vi "Sweep.vi"(0 "LINX Resource":T1, 5 "Bias V":dbl, 7 "steps to record":i32, 11 "error in (no error)":errorcluster) -> (4 "LINX Resource 2":T1, 6 "PD current (A)":dbl[](array[numeric]), 8 "Incidence angle (deg)":dbl[](array[numeric]), 10 "PD Voltage (V)":dbl[](array[numeric]), 15 "Error Out":errorcluster)   [LabVIEW 2020]
uses:
  <vilib>/MakerHub/LINX/Private/Type Defs/LINX Ref.ctl
  <vilib>/MakerHub/LINX/Private/Type Defs/Platform.ctl
  <vilib>/MakerHub/LINX/Private/Type Defs/Interface.ctl
  <vilib>/MakerHub/LINX/Private/Device/Type Defs/LINX Device Config.ctl
  <vilib>/MakerHub/LINX/Private/Device/Type Defs/TCP Config.ctl
  <vilib>/MakerHub/LINX/Private/Device/Type Defs/Channels.ctl
  <vilib>/MakerHub/LINX/Public/Peripherals/Digital/Digital Write 1 Chan.vi
  <vilib>/MakerHub/LINX/Public/Peripherals/Digital/Digital Write N Chans.vi
  <vilib>/MakerHub/LINX/Private/Local IO/LinxDigitalWrite.vi
  <vilib>/MakerHub/LINX/Public/Utilities/Check Channel.vi
  <vilib>/MakerHub/LINX/Private/Utilties/Generate Error.vi
  <vilib>/MakerHub/LINX/LMH-LINX.lvlib
  <vilib>/MakerHub/LINX/Private/Device/Device.lvlib
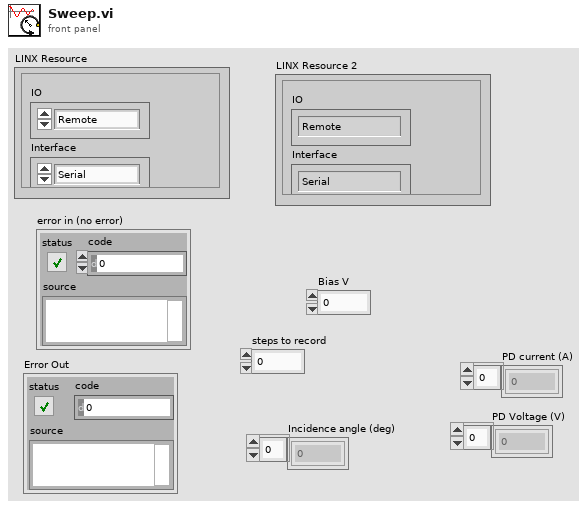
[diagram p1: front panel]
types:
  T1 = typedef "LMH-LINX.lvlib/LINX Ref.ctl" = cluster{"IO":T2, "Interface":T3, "LINX Device Config":T4}
  T2 = typedef "LMH-LINX.lvlib/Platform.ctl" = enum16{"Remote", "Local"}
  T3 = typedef "LMH-LINX.lvlib/Interface.ctl" = enum16{"Serial", "TCP"}
  T4 = typedef "LMH-LINX.lvlib/Device.lvlib/LINX Device Config.ctl" = cluster{"Interface":T3, "COM Port":refnum<visa-resource-name>, "TCP Configuration":T5, "Device Family":u8, "Device ID":u8, "Device Name":string, "TCP Ref":refnum<k5>, "Channels":T6}
  T5 = typedef "LMH-LINX.lvlib/Device.lvlib/TCP Config.ctl" = cluster{"IP Address":string, "Port":u16}
  T6 = typedef "LMH-LINX.lvlib/Channels.ctl" = cluster{"DI":u8[], "DO":u8[], "AI":u8[], "AO":u8[], "PWM":u8[], "QE":u8[], "UART":u8[], "I2C 2":u8[], "SPI":u8[], "CAN":u8[], "Servo":u8[], "AI Ref (V)":dbl, "AI Resolution (Bits)":u8, "AO Ref (V)":dbl, "AO Resolution (Bits)":u8}
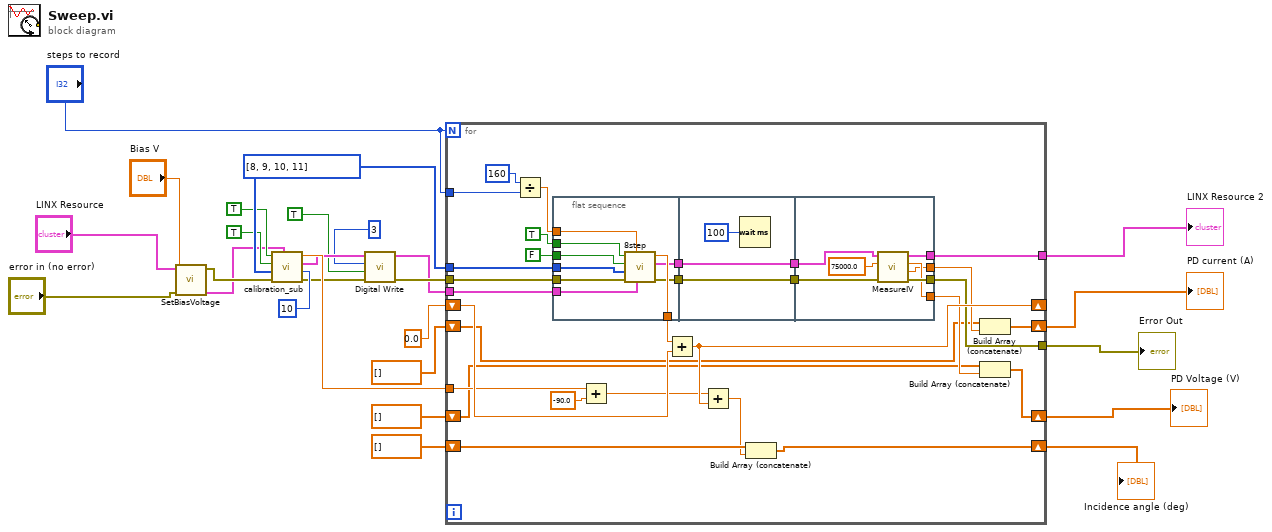
[diagram p0: block diagram]
diagram:
  w26 = u8[] [8, 9, 10, 11] ("DO Channels")
  n1 = call "SetBiasVoltage.vi"("Error In"="error in (no error)", "Bias V"="Bias V", "LINX Resource"="LINX Resource") -> ("LINX Resource 2"=w2:T1, "Error Out"=w3:errorcluster)  [unwired: 7 in]
  n2 = call "calibration_sub.vi"("Angle in"=10, "LINX Resource"=w2, "error in (no error)"=w3, "DO Channels"=w26, "CCW"=TRUE, "Start calibration"=TRUE) -> ("error out"=w13:errorcluster, "LINX Resource out"=w14:T1, "Actual angle out"=w21:dbl)  [unwired: 3 in]
  n3 = call-poly <vilib>:"Digital Write.vi"("Error In"=w13, "Output Value"=TRUE, "DO Channel"=u8 3, "LINX Resource"=w14) -> ("Error Out"=w12:errorcluster, "LINX Resource"=w11:T1)  [unwired: 6 in]
  n4 = for {
    N: "steps to record" -> [_]
    tunnel: "steps to record" -> [w54]
    shift-right: [w50] -> _
    shift-left: 0.0 -> [w53]
    tunnel: w26 -> [w42]
    tunnel: w11 -> [w44]
    tunnel: w21 -> [w52]
    shift-right: [w48] -> w6
    shift-left: dbl[] [] -> [w47]
    shift-right: [w45] -> w7
    shift-left: dbl[] [] -> [w30]
    tunnel: w12 -> [w36]
    tunnel: [w33] -> w25
    tunnel: [w32] -> w24
    shift-right: [w28] -> w8
    shift-left: dbl[] [] -> [w27]
    n5 = Divide(x=160 ("Angle in"), y=w54) -> (x/y=w43:dbl)
    n6 = flat-sequence {
      tunnel: w44 -> [w64]
      tunnel: w43 -> [w63]
      tunnel: w42 -> [w62]
      tunnel: FALSE ("CCW") -> [w61]
      tunnel: TRUE ("OK Button") -> [w60]
      tunnel: [w59] -> w39
      tunnel: [w58] -> w37
      tunnel: w36 -> [w57]
      tunnel: [w56] -> w34
      tunnel: [w66] -> w38
      tunnel: w37 -> [w66]
      tunnel: [w65] -> w35
      tunnel: w34 -> [w65]
      tunnel: w38 -> [w74]
      tunnel: w35 -> [w73]
      tunnel: [w72] -> w33
      tunnel: [w71] -> w32
      tunnel: [w69] -> w31
      tunnel: [w68] -> w29
      frame #0 {
        n7 = call "8step.vi"("LINX Resource in"=w64, "Angle in"=w63, "error in (no error)"=w57, "DO Channels"=w62, "CCW"=w61, "OK Button"=w60) -> ("error out"=w56:errorcluster, "LINX Resource out"=w58:T1, "Actual angle out"=w59:dbl)  [unwired: 3 in]
      }
      frame #1 {
        n8 = Wait (ms)(milliseconds to wait=u32 100) -> ()  [unwired: 1 out]
      }
      frame #2 {
        n9 = call "MeasureIV.vi"("Error In"=w73, "Rf"=75000.0, "LINX Resource"=w74) -> ("Error Out"=w71:errorcluster, "PD Current (A)"=w68:dbl, "PD Voltage (V)"=w69:dbl, "LINX Resource 2"=w72:T1)  [unwired: 5 in]
      }
    }
    n10 = Add(x=w52, y=-90.0) -> (x+y=w49:dbl)
    n11 = Add(x=w39, y=w53) -> (x+y=w50:dbl)
    n12 = Add(x=w49, y=w50) -> (x+y=w46:dbl)
    n13 = Build Array (concatenate)(w47, w46) -> (w48:dbl[])
    n14 = Build Array (concatenate)(w27, w29) -> (w28:dbl[])
    n15 = Build Array (concatenate)(w30, w31) -> (w45:dbl[])
  }
  "LINX Resource 2" <- w25
  "Error Out" <- w24
  "PD current (A)" <- w8
  "PD Voltage (V)" <- w7
  "Incidence angle (deg)" <- w6
